vi "Launch Async Event Handler.vi"(8 "error in (no error)":errorcluster, 11 "ExecAnchor in":refnum<class "ExecAnchor.lvclass">) -> (0 "error out":errorcluster, 3 "ExecAnchor out":refnum<class "ExecAnchor.lvclass">)   [LabVIEW 2020, in "ExecAnchor.lvclass"]
uses:
  ExecAnchor.lvclass
  Wait Async.vi
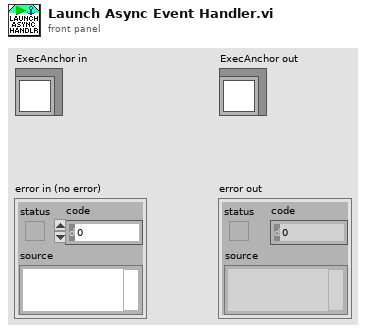
[diagram p1: front panel]
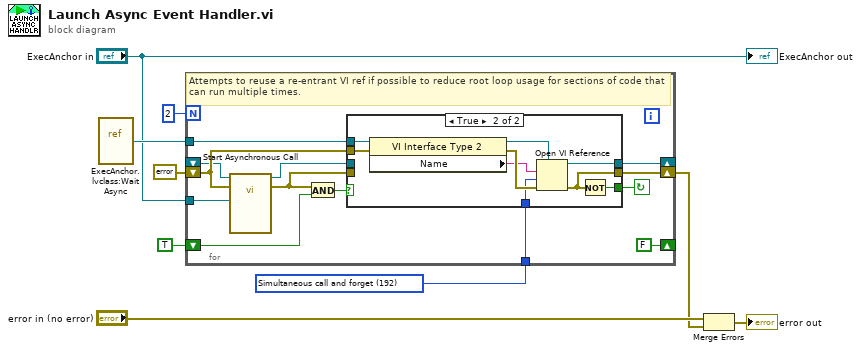
[diagram p0: block diagram]
diagram:
  w6 = 192 items=["Record modifications"=1, "Open templates for editing"=2, "Prompt user to save"=4, "Prepare for reentrant run"=8, "Prompt to find missing subVIs"=16, "Hide loading dialog box"=32, "Enable simultaneous calls"=64, "Prepare to call and forget"=128, "Simultaneous call and forget"=192, "Prepare to call and collect"=256, "Simultaneous call and collect"=320]
  n1 = vi-ref "ExecAnchor.lvclass:Wait Async.vi"() -> (w5:refnum<vi>)
  n2 = for {
    N: 2 -> [_]
    tunnel: w5 -> [w21]
    tunnel: w6 -> [w20]
    shift-right: [w19] -> _
    shift-left: _ -> [w18]
    shift-right: [w16] -> w2
    shift-left: errorcluster {"status"=FALSE, "code"=0, "source"=""} ("error constant") -> [w22]
    shift-right: [FALSE] -> _
    shift-left: TRUE -> [w13]
    tunnel: "ExecAnchor in" -> [w10]
    stop <- w12 continue-if-true
    # "Attempts to reuse a re-entrant VI ref if possible to reduce root loop usage for sections of code that can run multiple times."
    n3 = call-by-ref "Start Asynchronous Call"(reference=w18, error in=w22, "ExecAnchor in"=w10) -> (reference out=w17:refnum<vi>, error out=w15:errorcluster)  [unwired: 11 in]
    n4 = And(x=w15, y=w13) -> (x .and. y?=w14:bool)
    n5 = case shown="True" w14 {
      tunnel: w21 -> [_ w32]
      tunnel: w20 -> [_ w30]
      tunnel: [w24 w28] -> w19
      tunnel: w17 -> [w24 _]
      tunnel: [w23 w26] -> w16
      tunnel: w15 -> [w23 _]
      tunnel: w22 -> [_ w27]
      tunnel: [_ w25] -> w12
      frame False {
      }
      frame True {
        n6 = property class="VI Interface Type 2"(reference=w32, error in=w27) -> (reference out=w29:refnum<vi>, error out=w33:errorcluster, "Name"=w31:string)
        n7 = Open VI Reference(type specifier VI Refnum (for type only)=w29, vi path=w31, options=w30, error in (no error)=w33) -> (vi reference=w28:refnum<vi>, error out=w26:errorcluster)  [unwired: 2 in]
        n8 = Not(x=w26) -> (.not. x?=w25:bool)
      }
    }
  }
  n9 = Merge Errors("error in (no error)", w2) -> (→"error out":errorcluster)
  "ExecAnchor out" <- "ExecAnchor in"
